vi "UpdateLegParam.vi"(8 "error in (no error)":errorcluster) -> (0 "error out":errorcluster)   [LabVIEW 2016]
uses:
  Classes/CAlex2/TypeDef/LowerBodyDim.ctl
  Classes/ForceField/TypeDef/FF_Gains.ctl
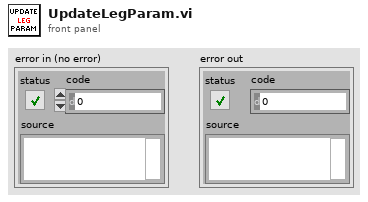
[diagram p1: front panel]
types:
  T1 = typedef "CAlex2.lvclass/LowerBodyDim.ctl" = cluster{"BodyDim":cluster{"ThighLt (m)":dbl, "ShankLt (m)":dbl, "HipWd (m)":dbl}, "BodyWt":cluster{"Thigh (kg)":dbl, "Shank (kg)":dbl}, "Cuff Loc":cluster{"HipCuffWd (m)":dbl, "HipCuffHt (m)":dbl, "HipFwdShift (m)":dbl, "ThighToKnee (m)":dbl, "ThighCuffDist (m)":dbl, "ShankToKnee (m)":dbl}}
  T2 = typedef "ForceField.lvclass/FF_Gains.ctl" = cluster{"Kn":dbl, "Dn":dbl, "Kt":dbl, "Dt":dbl, "Kd":dbl, "Ns":dbl}
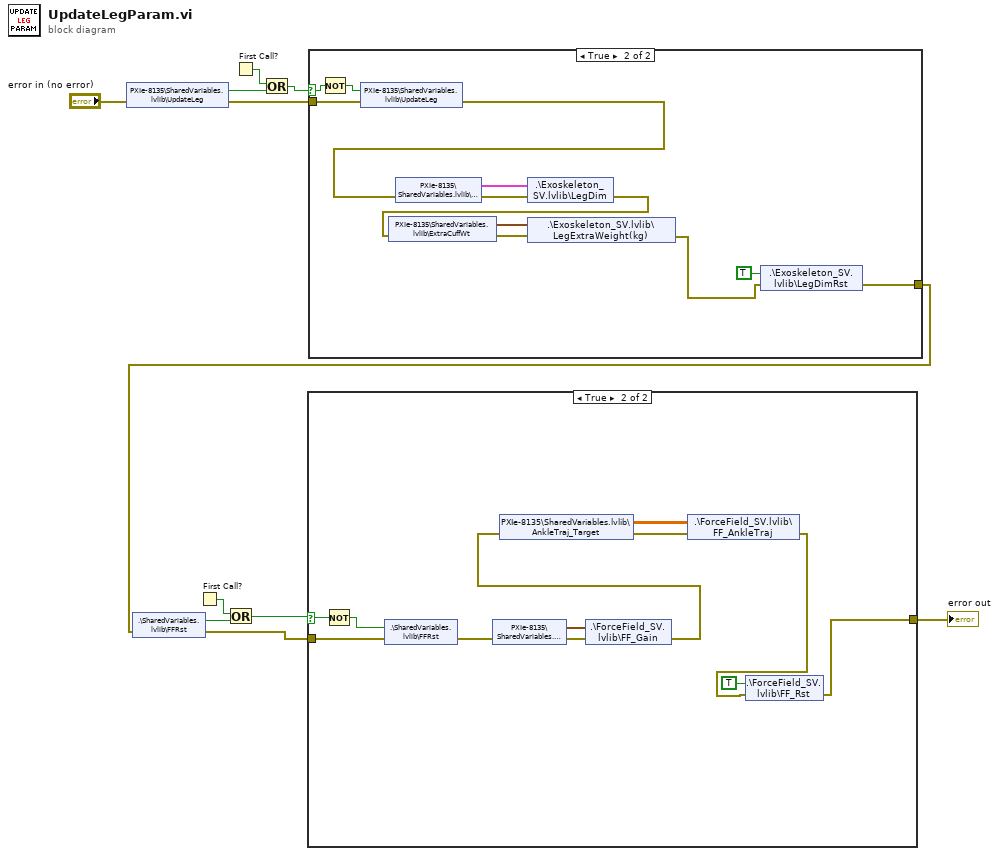
[diagram p0: block diagram]
diagram:
  n1 = shared-variable "PXIe-8135\\SharedVariables.lvlib\\UpdateLeg"(error in="error in (no error)") -> (w8:bool, error out=w11:errorcluster)
  n2 = First Call?() -> (First Call?: T/F=w6:bool)
  n3 = First Call?() -> (First Call?: T/F=w9:bool)
  n4 = Or(x=w9, y=w8) -> (x .or. y?=w7:bool)
  n5 = case shown="True" w7 {
    selector: w7 -> [_ w18]
    tunnel: w11 -> [w12 w24]
    tunnel: [w12 w19] -> w2
    frame False {
    }
    frame True {
      n6 = Not(x=w18) -> (.not. x?=w17:bool)
      n7 = shared-variable "PXIe-8135\\SharedVariables.lvlib\\UpdateLeg"(w17, error in=w24) -> (error out=w20:errorcluster)
      n8 = shared-variable "PXIe-8135\\SharedVariables.lvlib\\LegDim"(error in=w20) -> (w21:T1, error out=w23:errorcluster)
      n9 = shared-variable ".\\Exoskeleton_SV.lvlib\\LegDim"(w21, error in=w23) -> (error out=w16:errorcluster)
      n10 = shared-variable "PXIe-8135\\SharedVariables.lvlib\\ExtraCuffWt"(error in=w16) -> (w15:cluster{"Thigh":dbl, "Shank":dbl}, error out=w14:errorcluster)
      n11 = shared-variable ".\\Exoskeleton_SV.lvlib\\LegExtraWeight(kg)"(w15, error in=w14) -> (error out=w13:errorcluster)
      n12 = shared-variable ".\\Exoskeleton_SV.lvlib\\LegDimRst"(TRUE ("ResetArm"), error in=w13) -> (error out=w19:errorcluster)
    }
  }
  n13 = shared-variable ".\\SharedVariables.lvlib\\FFRst"(error in=w2) -> (w5:bool, error out=w3:errorcluster)
  n14 = Or(x=w6, y=w5) -> (x .or. y?=w4:bool)
  n15 = case shown="True" w4 {
    selector: w4 -> [_ w37]
    tunnel: w3 -> [w25 w35]
    tunnel: [w25 w30] -> w1
    frame False {
    }
    frame True {
      n16 = Not(x=w37) -> (.not. x?=w36:bool)
      n17 = shared-variable ".\\SharedVariables.lvlib\\FFRst"(w36, error in=w35) -> (error out=w34:errorcluster)
      n18 = shared-variable "PXIe-8135\\SharedVariables.lvlib\\Gains"(error in=w34) -> (w33:T2, error out=w32:errorcluster)
      n19 = shared-variable ".\\ForceField_SV.lvlib\\FF_Gain"(w33, error in=w32) -> (error out=w27:errorcluster)
      n20 = shared-variable "PXIe-8135\\SharedVariables.lvlib\\AnkleTraj_Target"(error in=w27) -> (w29:dbl[][], error out=w28:errorcluster)
      n21 = shared-variable ".\\ForceField_SV.lvlib\\FF_AnkleTraj"(w29, error in=w28) -> (error out=w26:errorcluster)
      n22 = shared-variable ".\\ForceField_SV.lvlib\\FF_Rst"(TRUE ("ResetArm"), error in=w26) -> (error out=w30:errorcluster)
    }
  }
  "error out" <- w1
